vi "Intake Command Handler.vi"(11 "Buttons":bool[](array[boolean])) -> ()   [LabVIEW 2019]
uses:
  Implementation/Intake Operations.ctl
panel:
  # "e"
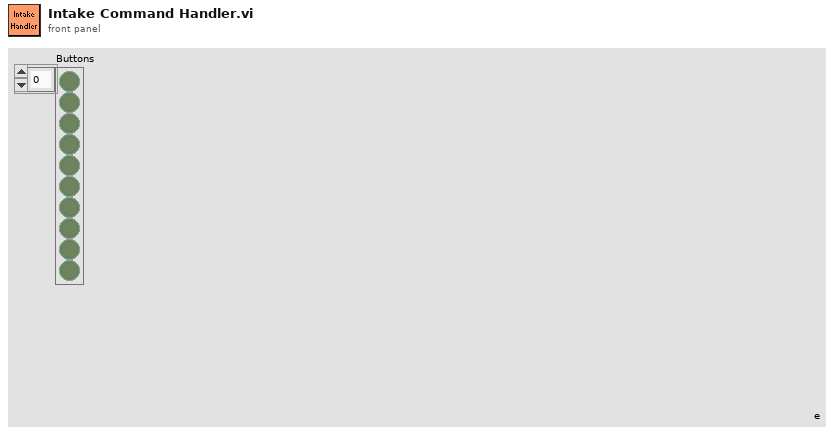
[diagram p1: front panel]
types:
  T1 = typedef "Intake Operations.ctl" = enum16{"Reserve", "Read Current", "Immediate", "Up", "Down"}
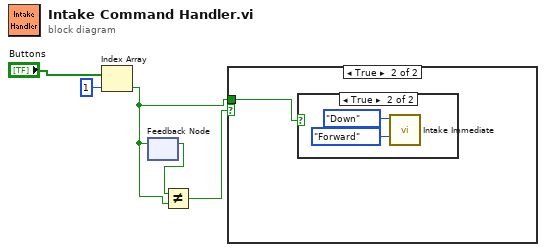
[diagram p0: block diagram]
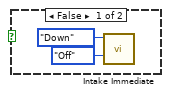
[diagram p3: hidden frame]
diagram:
  n1 = Index Array(array="Buttons", index=1) -> (element=w1:bool)
  n2 = feedback-in #1(w1) -> ()
  n3 = feedback #1() -> (w3:bool)  [unwired: 1 in]
  n4 = Not Equal?(x=w3, y=w1) -> (x != y?=w2:bool)
  n5 = case shown="True" w2 {
    tunnel: w1 -> [_ w6]
    frame False {
    }
    frame True {
      n6 = case shown="True" w6 {
        frame False {
          n7 = call "Intake Immediate.vi"("Rollers"=enum16{"Off", "Reverse", "Forward"}."Off", "Pivot"=Intake_Operations."Down") -> ()  [unwired: 9 in, 1 out]
        }
        frame True {
          n8 = call "Intake Immediate.vi"("Rollers"=enum16{"Off", "Reverse", "Forward"}."Forward", "Pivot"=Intake_Operations."Down") -> ()  [unwired: 9 in, 1 out]
        }
      }
    }
  }
